vi "TestExec.Read File Sync Type Option.vi"(8 "error in":errorcluster, 11 "Config File Path":path) -> (0 "error out":errorcluster, 3 "Diff(T)/All(F)":bool)   [LabVIEW 2018]
uses:
  <vilib>/Utility/config.llb/Read Key (String).vi
  <vilib>/Utility/config.llb/NI_LVConfig.lvlib
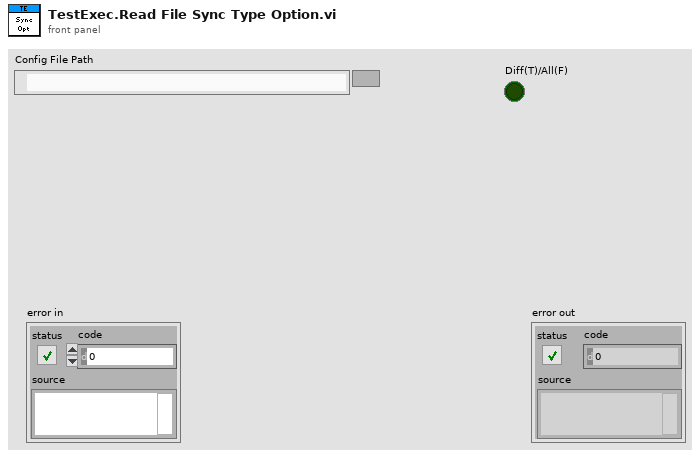
[diagram p1: front panel]
types:
  T1 = typedef "NI_LVConfig.lvlib/Config Data RefNum.ctl" = refnum<k1>
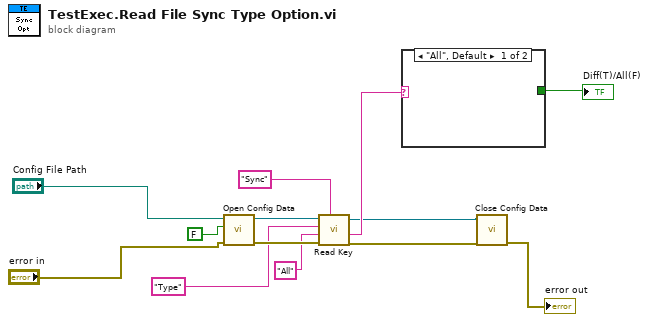
[diagram p0: block diagram]
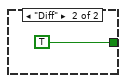
[diagram p2: hidden frame]
diagram:
  n1 = call <vilib>:"Open Config Data.vi"("error in (no error)"="error in", "create file if necessary (T)"=FALSE, "configuration file path"="Config File Path") -> ("error out"=w11:errorcluster, "refnum"=w12:T1)  [unwired: 6 in, 1 out]
  n2 = call-poly <vilib>:"Read Key.vi"("section"="Sync", "error in (no error)"=w11, "default value"="All", "key"="Type", "refnum"=w12) -> ("error out"=w1:errorcluster, "value"=w4:string, "refnum out"=w2:T1)  [unwired: 3 in, 1 out]
  n3 = case shown="\"All\", Default" w4 {
    tunnel: [_ TRUE] -> w3
    frame "All", Default {
    }
    frame "Diff" {
    }
  }
  "Diff(T)/All(F)" <- w3
  n4 = call <vilib>:"Close Config Data.vi"("error in (no error)"=w1, "refnum"=w2) -> ("error out"=→"error out":errorcluster)  [unwired: 8 in, 1 out]
